vi "Base_eleve (1).vi"() -> ()   [LabVIEW 2018]
uses:
  <vilib>/Instr/_visa.llb/VISA Configure Serial Port (Instr).vi
panel:
  in  "Chemin de fichier":path
  in  "Nom du fichier":string
  in  "Pause":bool
  in  "Enregistrer":bool
  out "Array 3":dbl[](array[numeric])
  out "Array 2":dbl[](array[numeric])
  out "Moy":dbl
  out "Moy":dbl
  out "Array":dbl[](array[numeric])
  out "Moy":dbl
  out "Min":dbl
  out "Max":dbl
  out "Min":dbl
  out "Max":dbl
  out "Min":dbl
  out "Max":dbl
  out "Temperature":dbl(graph)
  out "Pressure":dbl(graph)
  out "Humidity":dbl(graph)
  out "Temperature":dbl
  out "Pressure":dbl
  out "Humidity":dbl
  out "Chaîne":string
  in  "stop":bool
  in  "Nom de ressource VISA":refnum<visa-resource-name>
  # "1. Brancher la carte Arduino sur un port USB\n2. Choisir le port COM de la carte dans la liste déroulante \"Nom de ressource VISA\"\n3. Lancer le programme"
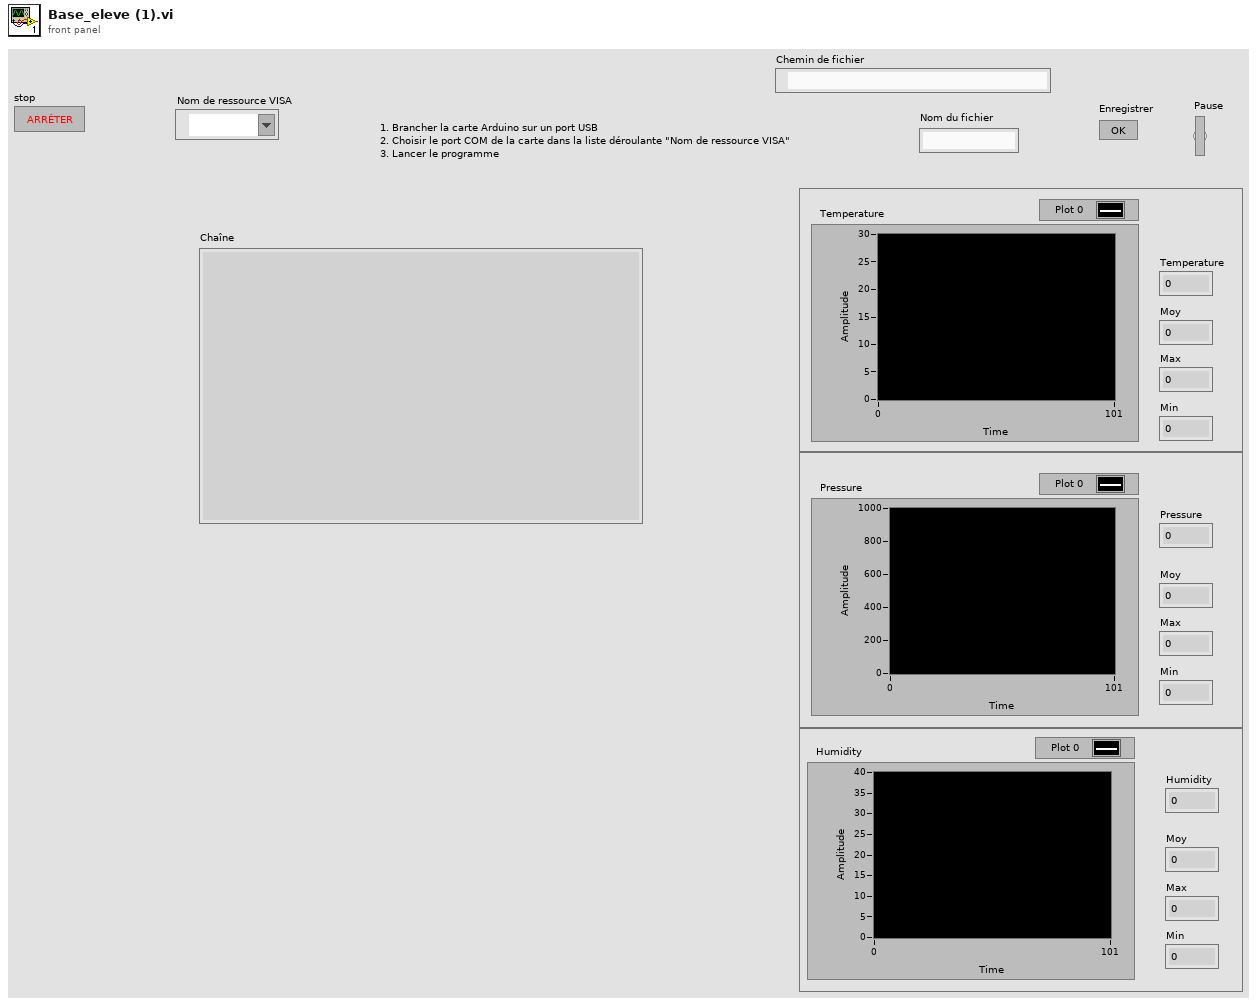
[diagram p1: front panel]
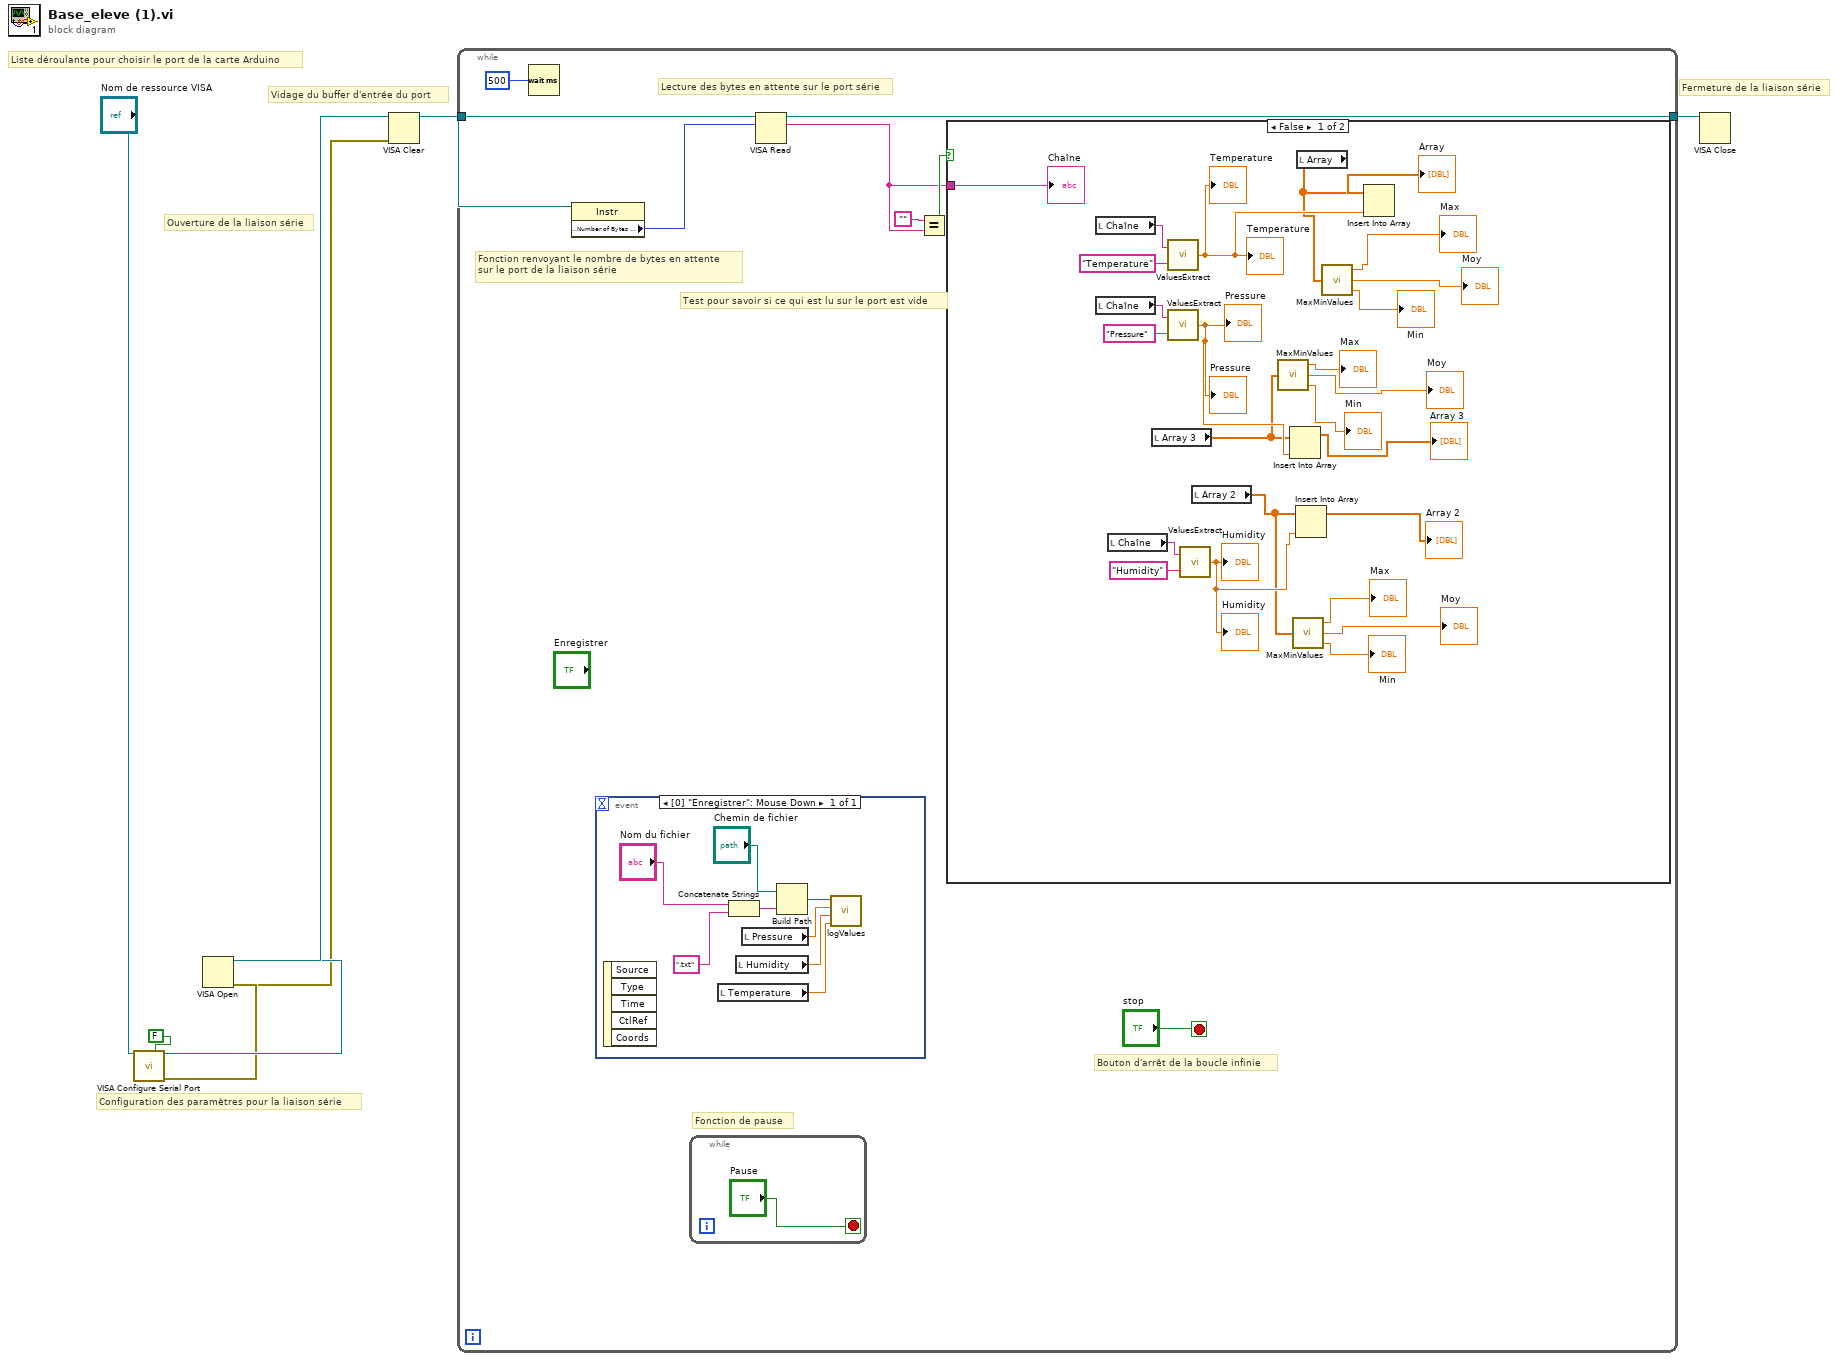
[diagram p0: block diagram]
diagram:
  # "Vidage du buffer d'entrée du port"
  # "Ouverture de la liaison série"
  # "Configuration des paramètres pour la liaison série"
  # "Liste déroulante pour choisir le port de la carte Arduino"
  # "Fermeture de la liaison série"
  n1 = call-poly "VISA Configure Serial Port"("VISA resource name"="Nom de ressource VISA", "Enable Termination\nChar (T)"=FALSE ("Enable Termination\nChar (T)")) -> ("VISA resource name out"=w5:refnum<visa-resource-name>, "error out"=w3:errorcluster)  [unwired: 12 in]
  n2 = VISA Open(error in (no error)=w3, VISA resource name=w5) -> (VISA resource name=w7:refnum<visa-resource-name>, error out=w2:errorcluster)  [unwired: 3 in]
  n3 = VISA Clear(VISA resource name=w7, error in (no error)=w2) -> (VISA resource name out=w6:refnum<visa-resource-name>)  [unwired: 1 out]
  n4 = while {
    tunnel: w6 -> [w15]
    tunnel: [w13] -> w1
    stop <- "stop" stop-if-true
    # "Fonction de pause"
    # "Lecture des bytes en attente sur le port série"
    # "Fonction renvoyant le nombre de bytes en attente\nsur le port de la liaison série"
    # "Test pour savoir si ce qui est lu sur le port est vide"
    # "Bouton d'arrêt de la boucle infinie"
    n5 = Wait (ms)(milliseconds to wait=u32 500 ("attente (ms)")) -> ()  [unwired: 1 out]
    n6 = property class="Instr"(reference=w15) -> ("Serial Settings:Number of Bytes at Serial Port"=w14:u32)  [unwired: 1 in, 2 out]
    n7 = event shown="[0] \"Enregistrer\": Mouse Down" {
      selector: _ -> [_]
      dyn-events: _ -> [_]
      timeout: _ -> [_]
      event "Enregistrer": Mouse Down {
        n8 = event-data() -> ()  [unwired: 1 in, 5 out]
        n9 = local read "Temperature"() -> (w21:dbl)
        n10 = Concatenate Strings("Nom du fichier", ".txt") -> (w17:string)
        n11 = local read "Humidity"() -> (w22:dbl)
        n12 = local read "Pressure"() -> (w23:dbl)
        n13 = Build Path(base path="Chemin de fichier", name or relative path=w17) -> (appended path=w24:path)
        n14 = call "logValues.vi"("Numeric 3"=w21, "Numeric 2"=w22, "Numeric"=w23, "appended path"=w24) -> ()
      }
    }
    n15 = while {
      stop <- "Pause" stop-if-true
    }
    n16 = VISA Read(VISA resource name=w15, byte count=w14) -> (VISA resource name out=w13:refnum<visa-resource-name>, read buffer=w9:string)  [unwired: 1 in, 2 out]
    n17 = Equal?(x="", y=w9) -> (x = y?=w10:bool)
    n18 = case shown="False" w10 {
      tunnel: w9 -> [w50 _]
      frame False {
        n19 = local read "Chaîne"() -> (w45:string)
        n20 = local read "Chaîne"() -> (w47:string)
        n21 = local read "Chaîne"() -> (w49:string)
        n22 = local read "Array 3"() -> (w30:dbl[])
        n23 = call "ValuesExtract.vi"("Indication de la valeure"="Temperature", "Chaine de caractères"=w45) -> ("Resulta"=w43:dbl)
        "Temperature" <- w43
        "Temperature" <- w43
        n24 = call "ValuesExtract.vi"("Indication de la valeure"="Pressure", "Chaine de caractères"=w47) -> ("Resulta"=w38:dbl)
        "Pressure" <- w38
        "Pressure" <- w38
        n25 = call "ValuesExtract.vi"("Indication de la valeure"="Humidity", "Chaine de caractères"=w49) -> ("Resulta"=w41:dbl)
        "Humidity" <- w41
        "Humidity" <- w41
        n26 = local read "Array 2"() -> (w26:dbl[])
        n27 = call "MaxMinValues.vi"("Array"=w30) -> ("Max"=→"Max":dbl, "Moy"=→"Moy":dbl, "Min"=→"Min":dbl)
        n28 = Insert Into Array(array=w30, new element=w38) -> (→"Array 3":dbl[])  [unwired: 1 in]
        n29 = call "MaxMinValues.vi"("Array"=w26) -> ("Max"=→"Max":dbl, "Moy"=→"Moy":dbl, "Min"=→"Min":dbl)
        n30 = Insert Into Array(array=w26, new element=w41) -> (→"Array 2":dbl[])  [unwired: 1 in]
        n31 = local read "Array"() -> (w36:dbl[])
        n32 = call "MaxMinValues.vi"("Array"=w36) -> ("Max"=→"Max":dbl, "Moy"=→"Moy":dbl, "Min"=→"Min":dbl)
        n33 = Insert Into Array(array=w36, new element=w43) -> (→"Array":dbl[])  [unwired: 1 in]
        "Chaîne" <- w50
      }
      frame True {
      }
    }
  }
  n34 = VISA Close(VISA resource name=w1) -> ()  [unwired: 1 in, 1 out]
